vi "Custom VISA Get Address.vi"(7 "Remove COM port descriptor from Ring permanently? (False)":bool, 8 "error in (no error)":errorcluster, 11 "VISA menu ref":refnum<vi>) -> (0 "error out":errorcluster, 3 "VISA address":refnum<visa-resource-name>)   [LabVIEW 2020, in "Get COM Descriptor.lvlib"]
doc: "Call this to extract VISA address from custom VISA Ring. It will remove COM port descriptor string from the Ring value to obtain valid VISA name. \nOptionally it can remove COM port descriptor string from the Ring element. This is useful to call e.g. before app stores control values to INI file at the exit so there are valid VISA names only.\n\nDetails: https://github.com/smaslan/get-com-descriptor"
uses:
  Get COM Descriptor.lvlib
  <vilib>/regexp/Match Regular Expression.xnode
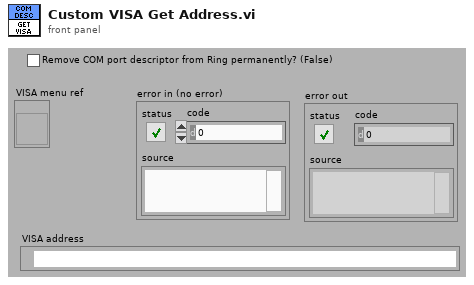
[diagram p1: front panel]
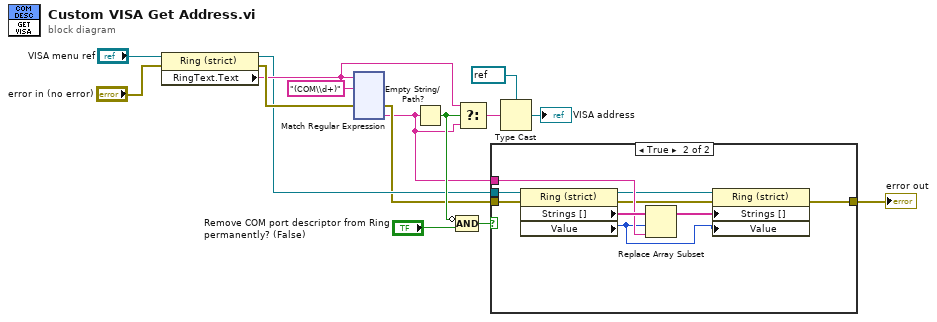
[diagram p0: block diagram]
diagram:
  n1 = property class="Ring (strict)"(reference="VISA menu ref", error in="error in (no error)") -> (reference out=w4:refnum<vi>, error out=w12:errorcluster, "RingText.Text"=w11:string)
  n2 = xnode "Match Regular Expression"("input string"=w11, "regular expression"="(COM\\d+)", "error in"=w12) -> ("error out"=w3:errorcluster, "submatch 1"=w2:string)  [unwired: 3 in, 4 out]
  n3 = Empty String/Path?(string/path=w2) -> (empty?=w7:bool)
  n4 = Compound Arithmetic op=AND(invert w7, "Remove COM port descriptor from Ring permanently? (False)") -> (w5:bool)
  n5 = Select(t=w11, s=w7, f=w2) -> (s? t:f=w9:string)
  n6 = case shown="True" w5 {
    tunnel: w4 -> [_ w25]
    tunnel: w3 -> [w16 w24]
    tunnel: w2 -> [_ w22]
    tunnel: [w16 w17] -> w1
    frame False {
    }
    frame True {
      n7 = property class="Ring (strict)"(reference=w25, error in=w24) -> (reference out=w21:refnum<vi>, error out=w20:errorcluster, "Strings []"=w23:string[], "Value"=w18:u16)
      n8 = Replace Array Subset(array=w23, new element=w22, index=w18) -> (w19:string[])
      n9 = property class="Ring (strict)"(reference=w21, error in=w20, "Strings []"=w19, "Value"=w18) -> (error out=w17:errorcluster)  [unwired: 1 out]
    }
  }
  "error out" <- w1
  n10 = Type Cast(type=refnum<visa-resource-name> refnum ("reference"), x=w9) -> (*(type *) &x=→"VISA address":refnum<visa-resource-name>)
